vi "Bool Utility.vi"(6 "Right Turn Lights":bool, 8 "Left Turn Lights":bool, 9 "Red Lights":bool, 10 "Headlights":bool, 11 "Values":bool[](array[boolean])) -> (3 "Values Out":bool[](array[boolean]))   [LabVIEW 2015]
panel:
  in  "Underr Lights":bool
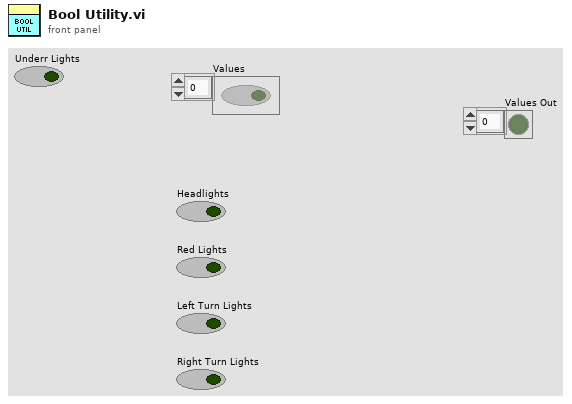
[diagram p1: front panel]
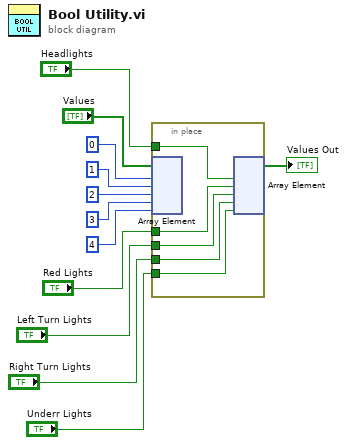
[diagram p0: block diagram]
diagram:
  n1 = in-place {
    in-place-border: "Headlights" -> [w17]
    in-place-border: "Red Lights" -> [w16]
    in-place-border: "Left Turn Lights" -> [w15]
    in-place-border: "Right Turn Lights" -> [w14]
    in-place-border: "Underr Lights" -> [w13]
    n2 = in-place-array #1("Values", 0, 1, 2, 3, 4) -> ()  [unwired: 5 out]
    n3 = in-place-array #1(w17, w16, w15, w14, w13) -> (→"Values Out":bool[])  [unwired: 5 out]
  }
